vi "Write Step Context.vi"(8 "error in (no error)":errorcluster, 10 "Step Context":T1={"StepIndex"=0, "Step"=refnum, "StartTime"=timestamp(0 s since 1904-01-01), "EndTime"=timestamp(0 s since 1904-01-01), "Result"=enum."Error", "Error Info"="", "Output Values"=[]}, 11 "Execution in":refnum<class "Execution.lvclass">) -> (0 "error out":errorcluster, 3 "Execution out":refnum<class "Execution.lvclass">)   [LabVIEW 2015, in "Execution.lvclass"]
uses:
  Execution.lvclass
  STEP_CONTEXT.ctl
  Step.lvclass
  Step/STEP_STATUS.ctl
  Execution.lvclass/Execution.ctl
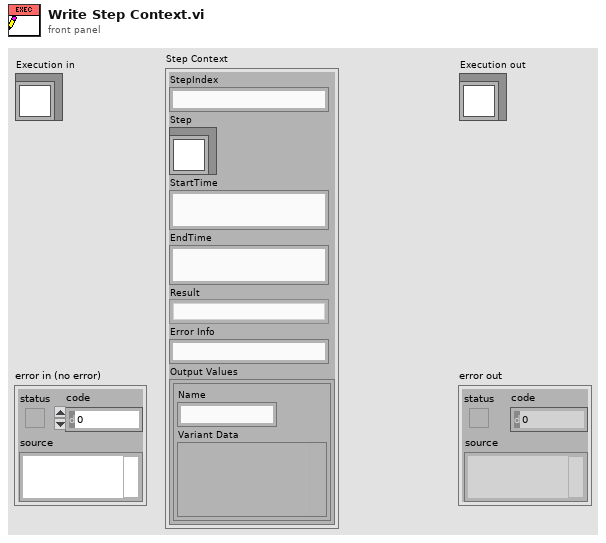
[diagram p1: front panel]
types:
  T1 = typedef "Execution.lvclass/STEP_CONTEXT.ctl" = cluster{"StepIndex":u32, "Step":refnum<class "Step.lvclass">, "StartTime":timestamp, "EndTime":timestamp, "Result":T2, "Error Info":string, "Output Values":cluster{"Name":string, "Variant Data":variant}[]}
  T2 = typedef "Step.lvclass/STEP_STATUS.ctl" = enum16{"Skipped", "Done", "Passed", "Failed", "Error"}
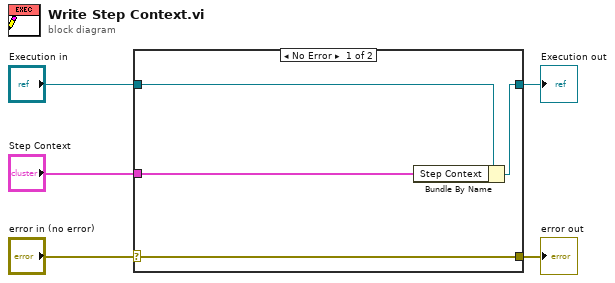
[diagram p0: block diagram]
diagram:
  n1 = case shown="No Error" "error in (no error)" {
    selector: "error in (no error)" -> [w9 w10]
    tunnel: [w9 w10] -> w4
    tunnel: [w7 w11] -> w2
    tunnel: "Execution in" -> [w8 w11]
    tunnel: "Step Context" -> [w6 _]
    frame No Error {
      n2 = Bundle By Name(cluster=w8, "Step Context"=w6) -> (w7:refnum<class "Execution.lvclass">)
    }
    frame Error {
    }
  }
  "error out" <- w4
  "Execution out" <- w2
